vi "To XML - When Branch is True - Adds XML Entities.vi"() -> ()   [LabVIEW 2017, in "Cobertura.Tests.lvlib" / "Line.lvlib"]
uses:
  Line.lvlib
  Cobertura/Line/Line.lvclass/Line.ctl
  Cobertura/Line/Write Branch.vi
  Cobertura/Line/Write Condition Coverage.vi
  <vilib>/xml/Close Reference(Node).vi
  Cobertura/Line/Line.lvclass
  <vilib>/xml/NI_XML.lvlib
  <resource>/objmgr/DOMUserDefRef.rc
  <vilib>/PNR/Transparent Assertions/Transparent Assertions/Transparent Assertions.lvlib
panel:
  out "error out":errorcluster
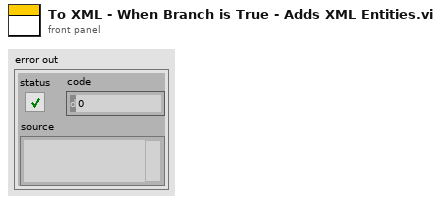
[diagram p1: front panel]
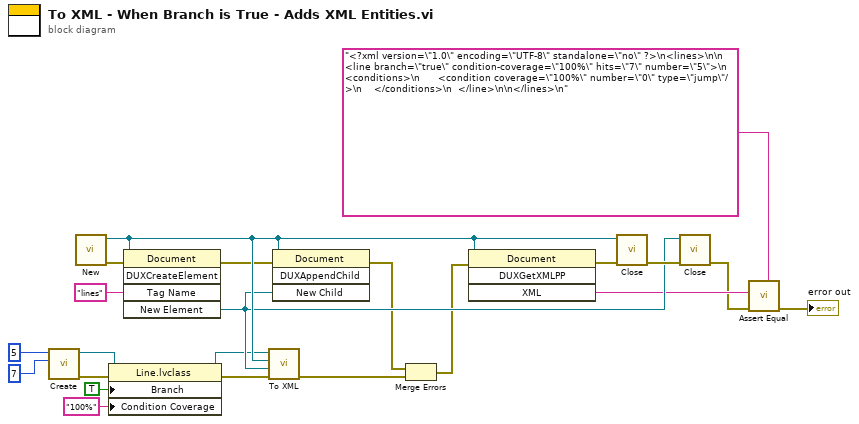
[diagram p0: block diagram]
diagram:
  n1 = call "Create.vi"("Hits"=u32 7, "Number"=u32 5) -> ("error out"=w22:errorcluster, "Line"=w4:refnum<class "Line.lvclass">)  [unwired: 8 in]
  n2 = call <vilib>:"New.vi"() -> ("error out"=w17:errorcluster, "DOM document out"=w19:refnum<k20>)  [unwired: 8 in]
  n3 = property class="Line.lvclass"(reference=w4, error in=w22, "Branch"=TRUE, "Condition Coverage"="100%") -> (reference out=w3:refnum<class "Line.lvclass">, error out=w5:errorcluster)
  n4 = invoke class="Document" method="DUXCreateElement"(reference=w19, error in=w17, "Tag Name"="lines") -> (error out=w18:errorcluster, "New Element"=w15:refnum<k20>)  [unwired: 2 in, 3 out]
  n5 = call-dynamic "To XML.vi"("error in (no error)"=w5, "Parent"=w15, "Document"=w19, "Line in"=w3) -> ("error out"=w7:errorcluster)  [unwired: 7 in]
  n6 = invoke class="Document" method="DUXAppendChild"(reference=w19, error in=w18, "New Child"=w15) -> (error out=w9:errorcluster)  [unwired: 1 in, 3 out]
  n7 = Merge Errors(w9, w7) -> (w8:errorcluster)
  n8 = invoke class="Document" method="DUXGetXMLPP"(reference=w19, error in=w8) -> (error out=w20:errorcluster, "XML"=w14:string)  [unwired: 2 in, 2 out]
  n9 = call-poly <vilib>:"Close.vi"("error in (no error)"=w20, "node"=w19) -> ("error out"=w16:errorcluster)  [unwired: 7 in]
  n10 = call-poly <vilib>:"Close.vi"("error in (no error)"=w16, "node"=w15) -> ("error out"=w6:errorcluster)  [unwired: 7 in]
  n11 = call <vilib>:"Assert Equal.vi"("Expected"="<?xml version=\"1.0\" encoding=\"UTF-8\" standalone=\"no\" ?>\n<lines>\n\n  <line branch=\"true\" condition-coverage=\"100%\" hits=\"7\" number=\"5\">\n    <conditions>\n      <condition coverage=\"100%\" number=\"0\" type=\"jump\"/>\n    </conditions>\n  </line>\n\n</lines>\n", "error in (no error)"=w6, "Actual"=w14) -> ("error out"=→"error out":errorcluster)  [unwired: 8 in]
